vi "Auto_corr.vi"(8 "m":i32=3, 9 "P":i32=9, 11 "input A":dbl[](array[numeric])=[1.0, 3.0, 5.0, 6.0, 1.0, 9.0, 0.0, 7.0, 4.0, 3.0, 9.0, 6.0, 1.0, 0.0, 0.0, 3.0, 8.0, 9.0, 2.0, 4.0, 5.0, 5.0, 1.0, 2.0, 0.0, 2.0, 3.0, 2.0, 1.0, 1.0, 0.0, 9.0, 8.0, 7.0, 4.0, 1.0, 1.0, 8.0, 9.0]) -> (0 "Sn":dbl[](array[numeric]), 3 "Acc":dbl[](array[numeric]))   [LabVIEW 2015]
panel:
  out "size(s)":i32
  out "ceil(x): smallest int >= x":dbl
  out "shift register":dbl[](array[numeric])
  out "Numeric":i32
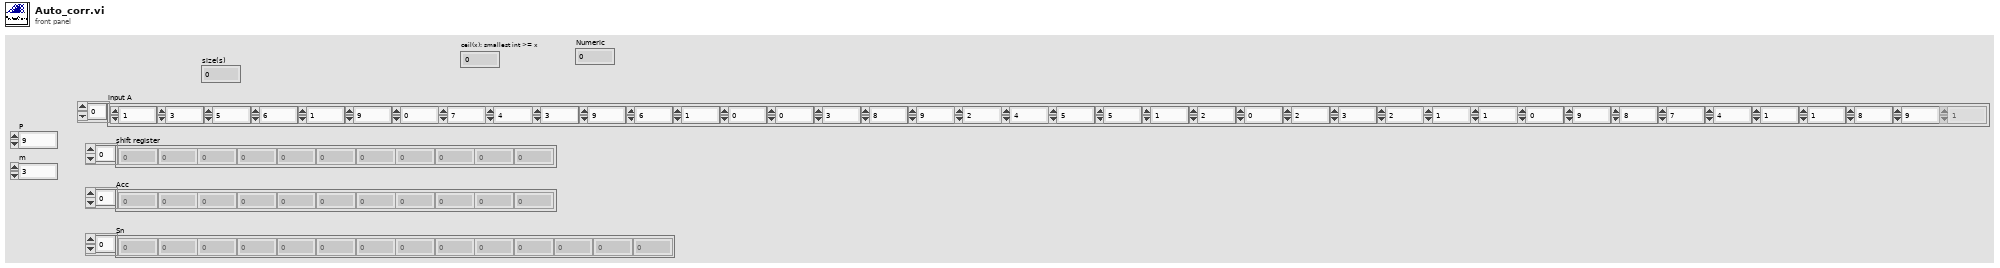
[diagram p1: front panel]
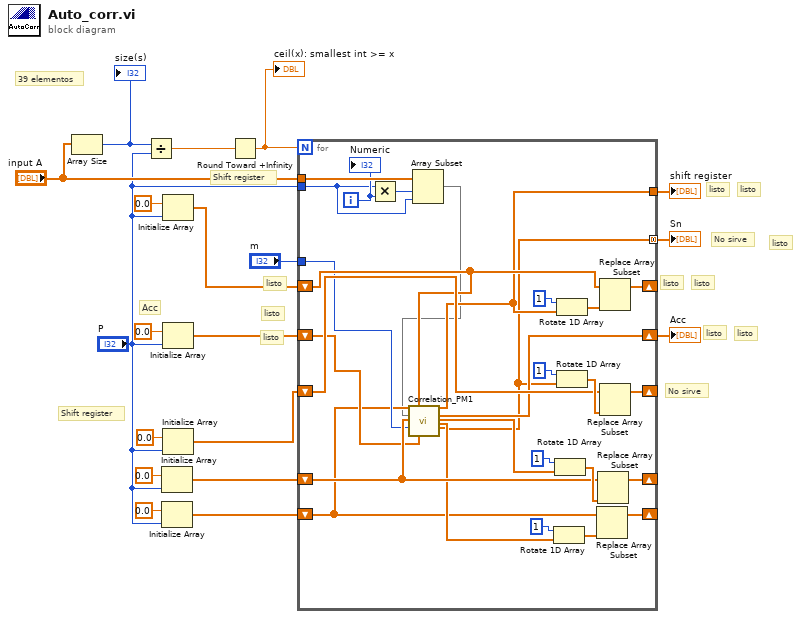
[diagram p0: block diagram]
diagram:
  # "No sirve"
  # "listo"
  # "listo"
  # "listo"
  # "listo"
  # "listo"
  # "listo"
  # "listo"
  # "No sirve"
  # "listo"
  # "listo"
  # "listo"
  # "Shift register"
  # "Acc"
  # "Shift register"
  # "39 elementos"
  n1 = Array Size(array="input A") -> (size(s)=w18:i32)
  "size(s)" <- w18
  n2 = Divide(x=w18, y="P") -> (x/y=w17:dbl)
  n3 = Initialize Array(0.0 ("dimension size"), "P") -> (w4:dbl[])
  n4 = Initialize Array(0.0 ("dimension size"), "P") -> (w2:dbl[])
  n5 = Initialize Array(0.0 ("dimension size"), "P") -> (w7:dbl[])
  n6 = Initialize Array(0.0 ("dimension size"), "P") -> (w6:dbl[])
  n7 = Initialize Array(0.0 ("dimension size"), "P") -> (w5:dbl[])
  n8 = Round Toward +Infinity(x=w17) -> (ceil(x): smallest int >= x=w16:dbl)
  "ceil(x): smallest int >= x" <- w16
  n9 = for {
    N: w16 -> [_]
    tunnel: "P" -> [w34]
    tunnel: "m" -> [w31]
    shift-right: [w45] -> _
    shift-left: w7 -> [w33]
    shift-right: [w23] -> w11
    shift-left: w6 -> [w30]
    tunnel: [w24] -> w15
    tunnel: "input A" -> [w44]
    tunnel: [w21] -> w10 mode=concatenating
    shift-right: [w40] -> _
    shift-left: w5 -> [w39]
    shift-right: [w36] -> _
    shift-left: w4 -> [w32]
    shift-right: [w27] -> _
    shift-left: w2 -> [w25]
    i -> [w35]
    n10 = Multiply(x=w34, y=w35) -> (x*y=w43:i32)
    n11 = Array Subset(array=w44, index=w43, length=w34) -> (w20:dbl[])
    n12 = call "Correlation_PM1.vi"("shift register D"=w25, "Input A"=w20, "shift register MY"=w32, "m"=w31, "shift register in"=w33, "Acc in"=w30) -> ("shift register"=w24:dbl[], "Acc"=w23:dbl[], "shift register Y out"=w22:dbl[], "shift register D out"=w26:dbl[], "MnA"=w21:dbl[])  [unwired: 17 in]
    n13 = Rotate 1D Array(1:w26, 2:1 ("n")) -> (0:w28:dbl[])
    n14 = Rotate 1D Array(1:w22, 2:1 ("n")) -> (0:w37:dbl[])
    n15 = Rotate 1D Array(1:w24, 2:1 ("n")) -> (0:w46:dbl[])
    n16 = Rotate 1D Array(1:w21, 2:1 ("n")) -> (0:w41:dbl[])
    n17 = Replace Array Subset(array=w25, new element=w28) -> (w27:dbl[])  [unwired: 1 in]
    n18 = Replace Array Subset(array=w32, new element=w37) -> (w36:dbl[])  [unwired: 1 in]
    n19 = Replace Array Subset(array=w33, new element=w46) -> (w45:dbl[])  [unwired: 1 in]
    n20 = Replace Array Subset(array=w39, new element=w41) -> (w40:dbl[])  [unwired: 1 in]
    "Numeric" <- w35
  }
  "shift register" <- w15
  "Acc" <- w11
  "Sn" <- w10
